vi "logical operators.vi"() -> ()   [LabVIEW 2024]
panel:
  out "s? t:f":string
  in  "Numeric 5":dbl
  in  "Numeric 4":dbl
  out "In Range?":bool
  out "coerced(x)":dbl
  in  "Numeric 3":dbl
  out "Boolean 3":bool
  in  "Numeric 2":dbl
  in  "Numeric":dbl
  out "x = y?":bool
  in  "Boolean 2":bool
  in  "Boolean":bool
  # "Number 1"
  # "Number 2"
  # "Number 4"
  # "Number 3"
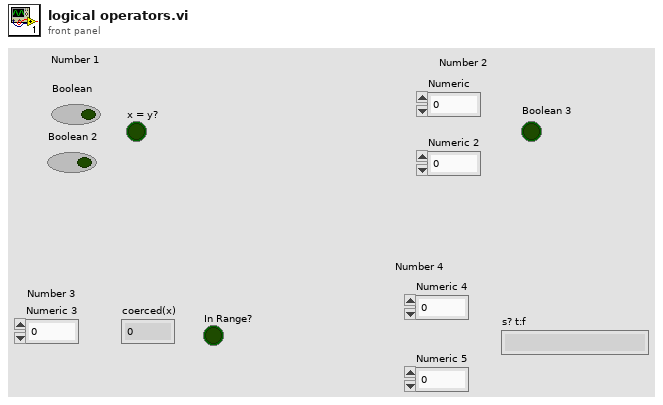
[diagram p1: front panel]
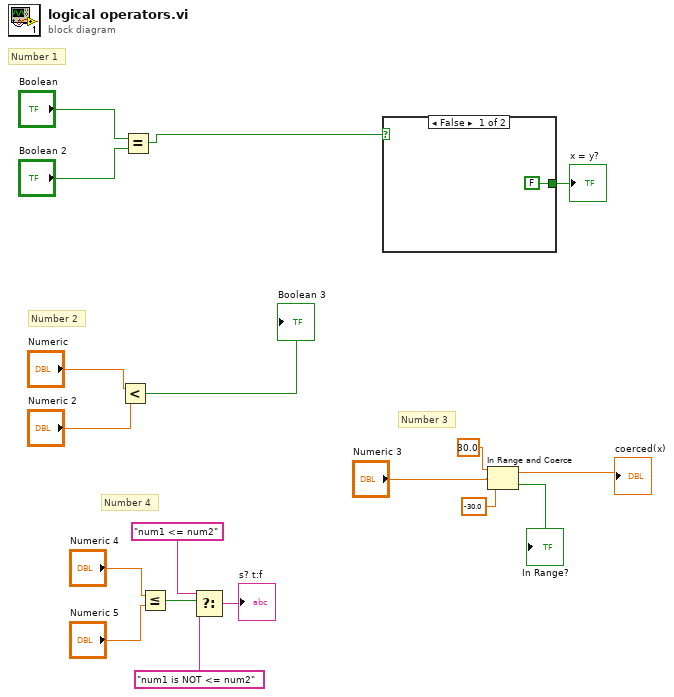
[diagram p0: block diagram]
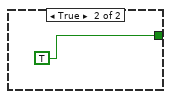
[diagram p2: hidden frame]
diagram:
  # "Number 4"
  # "Number 3"
  # "Number 2"
  # "Number 1"
  n1 = Less?(x="Numeric", y="Numeric 2") -> (x < y?=→"Boolean 3":bool)
  n2 = Equal?(x="Boolean", y="Boolean 2") -> (x = y?=w16:bool)
  n3 = Less Or Equal?(x="Numeric 4", y="Numeric 5") -> (x <= y?=w6:bool)
  n4 = Select(t="num1 <= num2", s=w6, f="num1 is NOT <= num2") -> (s? t:f=→"s? t:f":string)
  n5 = case shown="False" w16 {
    tunnel: [FALSE ("x = y?") TRUE ("x = y?")] -> w15
    frame False {
    }
    frame True {
    }
  }
  "x = y?" <- w15
  n6 = In Range and Coerce(upper limit=30.0, x="Numeric 3", lower limit=-30.0) -> (coerced(x)=→"coerced(x)":dbl, In Range?=→"In Range?":bool)
